vi "Self-Test.vi"(8 "error in (no error)":errorcluster, 11 "VISA resource name":refnum<visa-resource-name>) -> (0 "error out":errorcluster, 1 "Self-test message":string, 2 "Self test result":i32, 3 "VISA resource name out":refnum<visa-resource-name>)   [LabVIEW 2015, in "Rohde&Schwarz CMP LR WPAN Measurement.lvlib"]
doc: "This VI runs the instrument's self test routine and returns the test result. Some instruments can take a long time to perform the self-test, while some just return result of the self-test performed during the start-up.\n\nAttribute:\n-\n\nRemote-control command:\n*TST?"
uses:
  <instrlib>/Rohde&Schwarz CMP LR WPAN Measurement/Rohde&Schwarz CMP LR WPAN Measurement.lvlib
  <instrlib>/Rohde&Schwarz CMP LR WPAN Measurement/Private/rsidr_core.llb/type_Error_Codes.ctl
  <instrlib>/Rohde&Schwarz CMP LR WPAN Measurement/Private/rsidr_core.llb/rsidr_core.lvlib
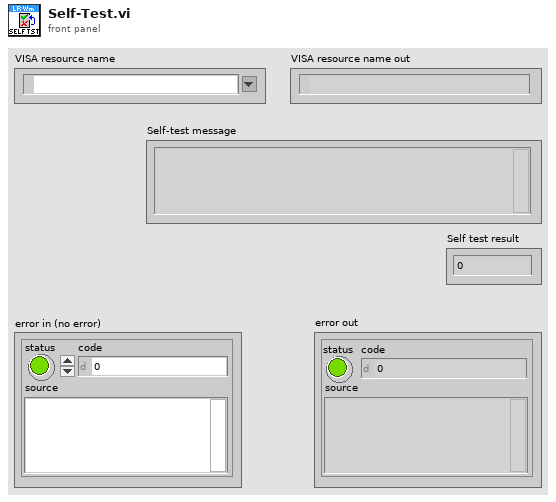
[diagram p1: front panel]
types:
  T1 = typedef "Rohde&Schwarz CMP LR WPAN Measurement.lvlib/rsidr_core.lvlib/type_Error_Codes.ctl" = enum16{"No_error", "VISA_err_ResourceNotFound", "VISA_err_Timeout", "VISA_warn_MoreDataAvailable", "RS_err_MissingCallback", "RS_err_InvalidAttribute", "RS_err_InvalidValue", "RS_err_UnknownResource", "RS_err_AlreadyInitialized", "RS_err_InstrumentStatus", "RS_err_BadRepCapName", "RS_err_TypesMismatch", "RS_err_ValueNotSupported", "RS_err_InvalidRngTable", "RS_err_IDqueryFail", "RS_err_UnexpResponse", "VISA_warn_ConfigNotLoaded", "RS_err_AttributeNotReadable", "RS_err_AttributeNotWritable", "RS_err_InstrumentType", "RS_err_InstrumentOption", "VISA_err_InvalidSize", "RS_err_ReliabilityIndicator", "VISA_warn_UnknownStatus", "VISA_warn_TermCharRead", "VISA_err_IO_error", "RS_err_FunctionNotSupported", "VISA_warn_QueueEmpty"}
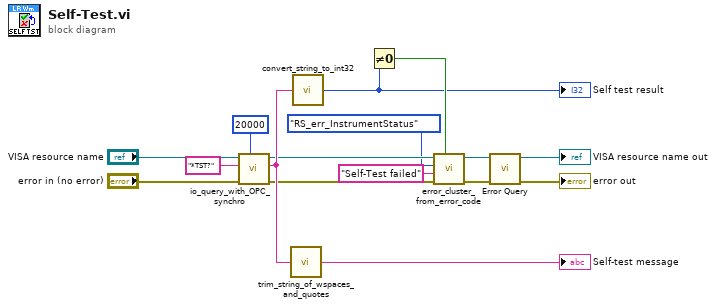
[diagram p0: block diagram]
diagram:
  n1 = call <instrlib>:"io_query_with_OPC_synchro.vi"("Timeout in (0 = OPC timeout)"=20000, "error in"="error in (no error)", "write buffer"="*TST?" ("Self-Test Command"), "VISA resource name"="VISA resource name") -> ("error out"=w14:errorcluster, "read buffer"=w15:string, "VISA resource name out"=w13:refnum<visa-resource-name>)  [unwired: 5 in]
  n2 = call <instrlib>:"trim_string_of_wspaces_and_quotes.vi"("String in"=w15) -> ("String out"=→"Self-test message":string)  [unwired: 4 in]
  n3 = call <instrlib>:"convert_string_to_int32.vi"("String in"=w15) -> ("int32 value out"=w4:i32)  [unwired: 4 in]
  "Self test result" <- w4
  n4 = Not Equal To 0?(x=w4) -> (x != 0?=w9:bool)
  n5 = call <instrlib>:"error_cluster_from_error_code.vi"("Error Creation Enabled (True)"=w9, "error in"=w14, "Error Message (\"\")"="Self-Test failed" ("error message (\"\")"), "Error Enum in"=type_Error_Codes."RS_err_InstrumentStatus", "VISA resource name"=w13) -> ("error out"=w12:errorcluster, "VISA resource name out"=w11:refnum<visa-resource-name>)  [unwired: 5 in]
  n6 = call <instrlib>:"Error Query.vi"("error in (no error)"=w12, "VISA resource name"=w11) -> ("error out"=→"error out":errorcluster, "VISA resource name out"=→"VISA resource name out":refnum<visa-resource-name>)  [unwired: 6 in, 2 out]
